vi "AlliGator Update Phasor Plot Image Overlay.vi"(7 "Image Control Refnum":T1 caption="Phasor Plot Display Refnum", 8 "error in (no error)":errorcluster, 9 "Overlay List":string[](array[string]), 11 "Phasor Plot Image in":T2) -> (0 "error out":errorcluster, 3 "Phasor Plot Image out":T2)   [LabVIEW 2021, in "AlliGator Phasor Plot.lvlib"]
doc: "Updates user-selected Phasor Plot image overlays."
uses:
  AlliGator Phasor Plot.lvlib
  <vilib>/vision/Image Controls.llb/IMAQ Image.ctl
  Image/Image Control Refnum.ctl
  <userlib>/_OpenG.lib/array/array.llb/Filter 1D Array (String)__ogtk.vi
  Time/Time.lvlib
  AlliGator Phasor Plot Color Map.lvlib
  <userlib>/_OpenG.lib/array/array.llb/openg_array.lvlib
  Image/Image.lvlib
panel:
  out "CPU (s)":dbl
  # "see the AlliGator License on the block diagram (Ctrl+E or Window:Show Block Diagram)"
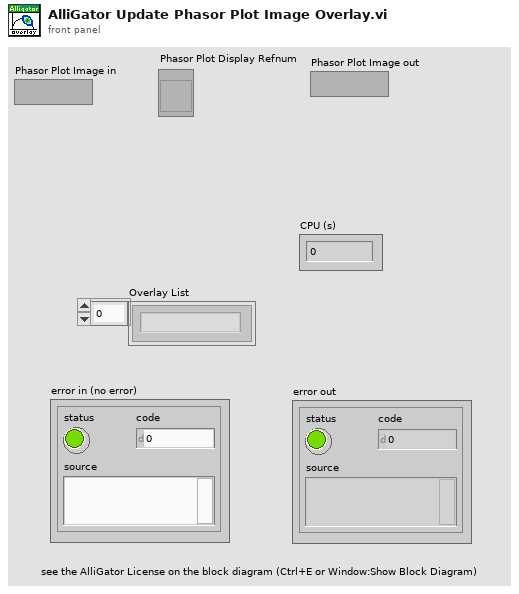
[diagram p1: front panel]
types:
  T1 = typedef "Image.lvlib/Image Control Refnum.ctl" = refnum<vi>
  T2 = typedef "IMAQ Image.ctl" = refnum<image>
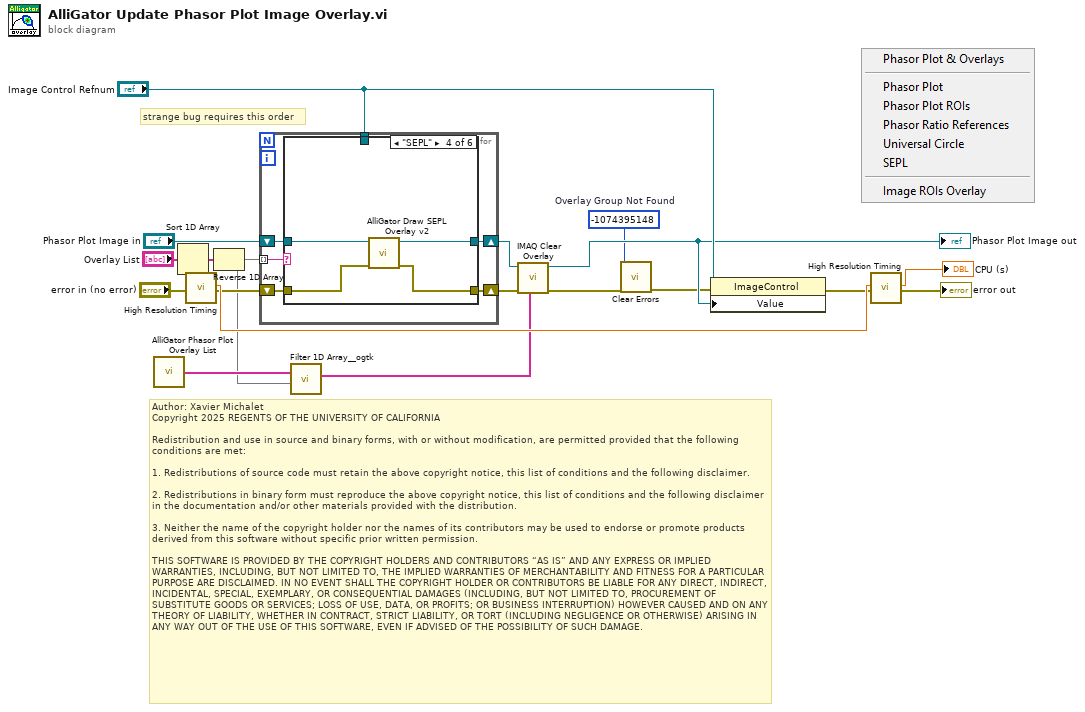
[diagram p0: block diagram]
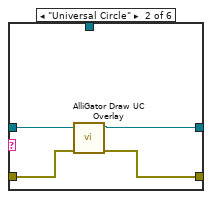
[diagram p3: hidden frame]
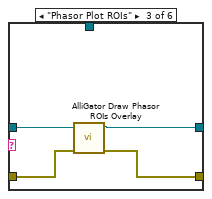
[diagram p4: hidden frame]
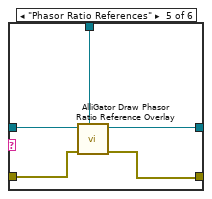
[diagram p5: hidden frame]
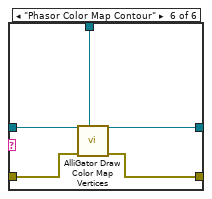
[diagram p6: hidden frame]
diagram:
  w1 = -1074395148  # Overlay Group Not Found
  # "Author: Xavier Michalet\nCopyright 2025 REGENTS OF THE UNIVERSITY OF CALIFORNIA\n\nRedistribution and use in source and binary forms, with or without modification, are permitted provided that the following conditions are met:\n\n1. Redistributions of source code must retain the above copyright notice, this list of conditions and the following disclaimer.\n\n2. Redistributions in binary form must reproduce the above copyright notice, this list of conditions and the following disclaimer in the documentation and/or other materials provided with the distribution.\n\n3. Neither the name of the copyright holder nor the names of its contributors may be used to endorse or promote products derived from this software without specific prior written permission.\n\nTHIS SOFTWARE IS PROVIDED BY THE COPYRIGHT HOLDERS AND CONTRIBUTORS “AS IS” AND ANY EXPRESS OR IMPLIED WARRANTIES, INCLUDING, BUT NOT LIMITED TO, THE IMPLIED WARRANTIES OF MERCHANTABILITY AND FITNESS FOR A PARTICULAR PURPOSE ARE DISCLAIMED. IN NO EVENT SHALL THE COPYRIGHT HOLDER OR CONTRIBUTORS BE LIABLE FOR ANY DIRECT, INDIRECT, INCIDENTAL, SPECIAL, EXEMPLARY, OR CONSEQUENTIAL DAMAGES (INCLUDING, BUT NOT LIMITED TO, PROCUREMENT OF SUBSTITUTE GOODS OR SERVICES; LOSS OF USE, DATA, OR PROFITS; OR BUSINESS INTERRUPTION) HOWEVER CAUSED AND ON ANY THEORY OF LIABILITY, WHETHER IN CONTRACT, STRICT LIABILITY, OR TORT (INCLUDING NEGLIGENCE OR OTHERWISE) ARISING IN ANY WAY OUT OF THE USE OF THIS SOFTWARE, EVEN IF ADVISED OF THE POSSIBILITY OF SUCH DAMAGE."
  # "strange bug requires this order"
  n1 = call "AlliGator Phasor Plot Overlay List.vi"() -> ("Phasor Plot Overlay List"=w9:string[])
  n2 = Sort 1D Array(array="Overlay List") -> (sorted array=w12:string[])
  n3 = call "High Resolution Timing.vi"("Error In"="error in (no error)") -> ("elapsed (relative) seconds"=w17:dbl, "Error Out"=w14:errorcluster)  [unwired: 16 in, 1 out]
  n4 = Reverse 1D Array(array=w12) -> (reversed array=w8:string[])
  n5 = for {
    shift-right: [w24] -> w6
    shift-left: "Phasor Plot Image in" -> [w25]
    shift-right: [w23] -> w7
    shift-left: w14 -> [w22]
    tunnel: w8 -> [w21] mode=indexing
    tunnel: "Image Control Refnum" -> [w20]
    n6 = case shown="\"SEPL\"" w21 {
      tunnel: w25 -> [w27 w31 w35 w39 w44 w49]
      tunnel: [w27 w30 w34 w38 w43 w48] -> w24
      tunnel: [w26 w28 w32 w36 w41 w46] -> w23
      tunnel: w22 -> [w26 w29 w33 w37 w42 w47]
      tunnel: w20 -> [_ _ _ _ w40 w45]
      frame "", Default {
        # "Phasor Plot ROIs case missing"
      }
      frame "Universal Circle" {
        n7 = call "AlliGator Draw UC Overlay.vi"("error in (no error)"=w29, "Refnum in"=w31) -> ("error out"=w28:errorcluster, "Refnum out"=w30:T2)  [unwired: 8 in]
      }
      frame "Phasor Plot ROIs" {
        n8 = call "AlliGator Draw Phasor ROIs Overlay.vi"("error in (no error)"=w33, "Refnum in"=w35) -> ("error out"=w32:errorcluster, "Refnum out"=w34:T2)  [unwired: 8 in]
      }
      frame "SEPL" {
        n9 = call "AlliGator Draw SEPL Overlay v2.vi"("error in (no error)"=w37, "Refnum in"=w39) -> ("error out"=w36:errorcluster, "Refnum out"=w38:T2)  [unwired: 8 in]
      }
      frame "Phasor Ratio References" {
        n10 = call "AlliGator Draw Phasor Ratio Reference Overlay.vi"("Image Control Refnum"=w40, "error in (no error)"=w42, "Phasor Plot Image in"=w44) -> ("error out"=w41:errorcluster, "Phasor Plot Image out"=w43:T2)  [unwired: 7 in]
      }
      frame "Phasor Color Map Contour" {
        n11 = call "AlliGator Draw Color Map Vertices.vi"("Image Control Refnum"=w45, "error in (no error)"=w47, "Phasor Plot Refnum in"=w49) -> ("error out"=w46:errorcluster, "Phasor Plot Refnum out"=w48:T2)  [unwired: 7 in]
      }
    }
  }
  n12 = call-poly <userlib>:"Filter 1D Array__ogtk.vi"("items to filter"=w8, "array"=w9) -> ("filtered array"=w4:string[])  [unwired: 4 in, 1 out]
  n13 = call "IMAQ Clear Overlay"("Groups"=w4, "error in (no error)"=w7, "Image"=w6) -> ("error out"=w3:errorcluster, "Image Out"=w5:T2)  [unwired: 7 in]
  "Phasor Plot Image out" <- w5
  n14 = call <vilib>:"Clear Errors.vi"("error in (no error)"=w3, "specific error code to clear (0: all)"=w1) -> ("error out"=w2:errorcluster)  [unwired: 4 in, 1 out]
  n15 = property class="ImageControl"(reference="Image Control Refnum", error in=w2, "Value"=w5) -> (error out=w11:errorcluster)  [unwired: 1 out]
  n16 = call "High Resolution Timing.vi"("relative seconds (NaN)"=w17, "Error In"=w11) -> ("elapsed (relative) seconds"=→"CPU (s)":dbl, "Error Out"=→"error out":errorcluster)  [unwired: 15 in, 1 out]
